vi "Col_Sum.vi"(0 "Image_2d":i16[][](array[numeric]), 5 "error in (no error)":errorcluster) -> (14 "Col_Sum":i16[](array[numeric]), 19 "error out":errorcluster)   [LabVIEW 2016]
panel:
  out "Waveform Graph":i16[](graph)
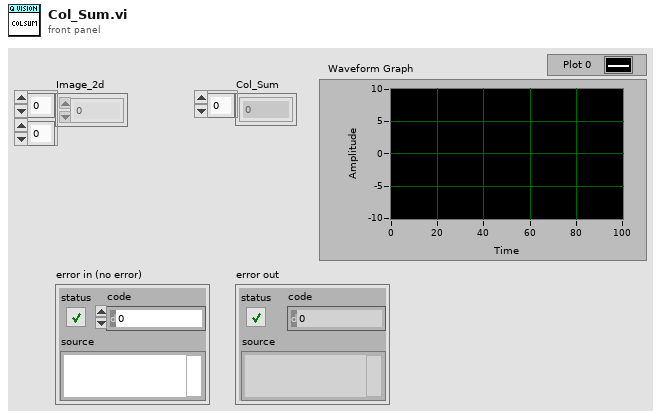
[diagram p1: front panel]
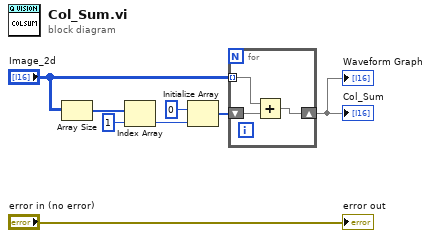
[diagram p0: block diagram]
diagram:
  n1 = Array Size(array="Image_2d") -> (size(s)=w3:i32[])
  n2 = Index Array(array=w3, index=1) -> (element=w5:i32)
  n3 = Initialize Array(i16 0 ("element"), w5) -> (w4:i16[])
  n4 = for {
    tunnel: "Image_2d" -> [w10] mode=indexing
    shift-right: [w9] -> w1
    shift-left: w4 -> [w11]
    n5 = Add(x=w10, y=w11) -> (x+y=w9:i16[])
  }
  "Col_Sum" <- w1
  "Waveform Graph" <- w1
  "error out" <- "error in (no error)"
